vi "Set Acquisition Channels.vi"(7 "Client parameters":cluster{"IP":string, "Port":u16}={"IP"="28.0.0.0", "Port"=6666}, 8 "Error In":errorcluster, 10 "Acquisition channels":T1, 11 "connection ID":refnum<k16>) -> (0 "Error Out":errorcluster, 3 "connection ID out":refnum<k16>)   [LabVIEW 2016, in "MKR1000.lvlib"]
doc: "This VI sets the channels to be acquired (0 to 5). Multiple channel can be acquired at the same time.\nThe VI try 5 times to receive ACKnowledgment for the sent command before returning Error 5000.\n\nNOTE:\nThe MKR1000 VI Library uses UDP. UDP is a connectionless protocol. With the term \"connection\" is intended that MKR1000 gives back an ACKnoledgment packet for each command sent. If no packet is returned (MKR1000 not connected to the net, out of range, etc.), the command is intended LOST and the VIs attempts to send the command again few times before returning Error 5000"
uses:
  MKR1000.lvlib
  Typedef/Set channels.ctl
  Typedef/MKR1000 - Commands.ctl
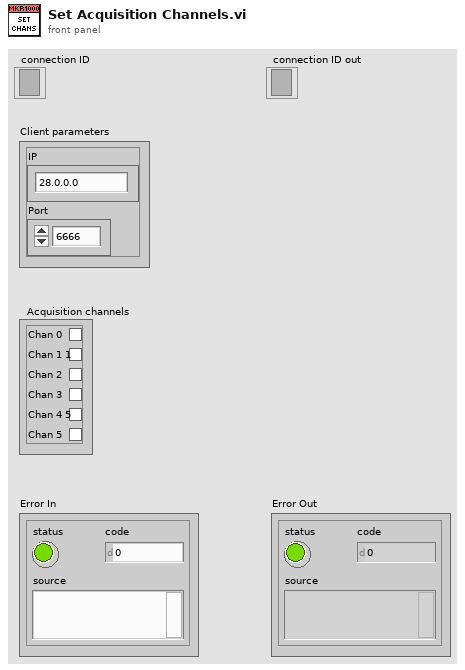
[diagram p1: front panel]
types:
  T1 = typedef "MKR1000.lvlib/Set channels.ctl" = cluster{"Chan 0":bool, "Chan 1 1":bool, "Chan 2":bool, "Chan 3":bool, "Chan 4 5":bool, "Chan 5":bool}
  T2 = typedef "MKR1000.lvlib/MKR1000 - Commands.ctl" = string
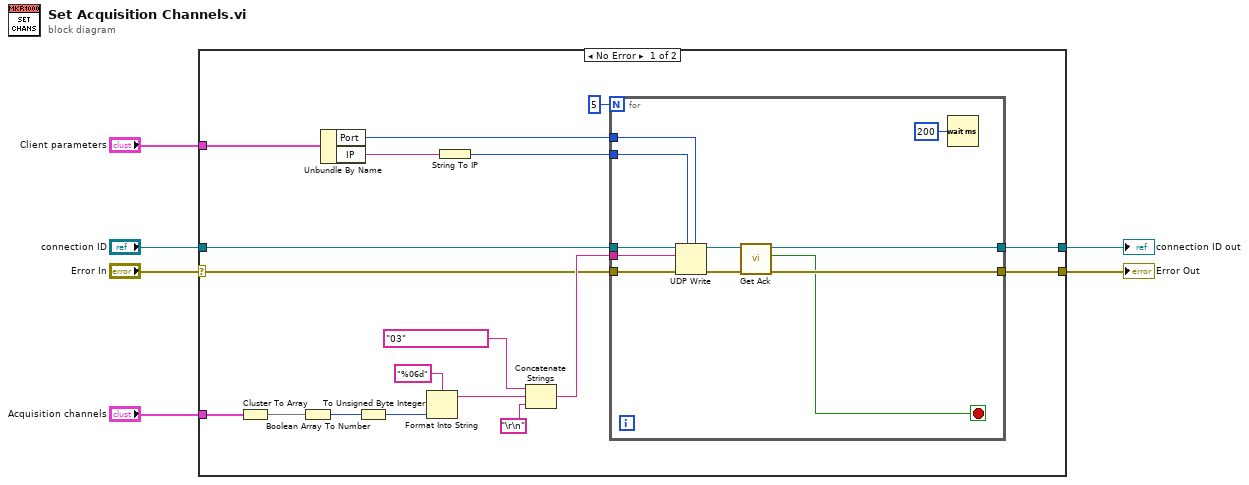
[diagram p0: block diagram]
diagram:
  n1 = case shown="No Error" "Error In" {
    selector: "Error In" -> [w14 w37]
    tunnel: "Acquisition channels" -> [w23 _]
    tunnel: "connection ID" -> [w21 w36]
    tunnel: "Client parameters" -> [w20 _]
    tunnel: [w8 w37] -> w2
    tunnel: [w9 w36] -> w1
    frame No Error {
      n2 = Cluster To Array(cluster=w23) -> (array=w22:bool[])
      n3 = Boolean Array To Number(Boolean array=w22) -> (number=w15:u32)
      n4 = Unbundle By Name(w20) -> ("Port"=w18:u16, "IP"=w19:string)
      n5 = To Unsigned Byte Integer(number=w15) -> (unsigned 8bit integer=w11:u8)
      n6 = Format Into String(format string="%06d", w11) -> (resulting string=w10:string)  [unwired: 2 in, 1 out]
      n7 = String To IP(1:w19) -> (0:w24:u32)
      n8 = Concatenate Strings(T2 "03" ("Combo Box"), w10, "\r\n") -> (w16:string)
      n9 = for {
        N: 5 -> [_]
        tunnel: w24 -> [w35]
        tunnel: w21 -> [w34]
        tunnel: w18 -> [w33]
        tunnel: w16 -> [w32]
        tunnel: w14 -> [w31]
        tunnel: [w29] -> w9
        tunnel: [w27] -> w8
        stop <- w26 stop-if-true
        n10 = UDP Write(address=w35, port or service name=w33, connection ID=w34, data in=w32, 8:w31) -> (error out=w28:errorcluster, 3:w30:refnum<k16>)  [unwired: 1 in]
        n11 = call "Get Ack.vi"("Error In"=w28, "connection ID"=w30) -> ("Error Out"=w27:errorcluster, "Ack status"=w26:bool, "connection ID out"=w29:refnum<k16>)  [unwired: 7 in]
        n12 = Wait (ms)(milliseconds to wait=u32 200) -> ()  [unwired: 1 out]
      }
    }
    frame Error {
    }
  }
  "Error Out" <- w2
  "connection ID out" <- w1
